vi "Debug - TCP - Write to Log File.vi"(9 "Transmission Log (or IP and Port String)":string, 10 "Flattened TCP Reference":string, 11 "Type of Write Opperation":T1) -> ()   [LabVIEW 2017, in "Communications Library.lvlib"]
doc: "Add a line to the TCP debug log file or modifys an already existing line to include the IP and Port number.\n\nWhen adding a new line, the placeholder should be used to mark the location where the IP and Port number will later be writte.\n\nNote: This VI must be non-reentrant, in order to avoid simulatenous writes to the same file by multiple threads."
uses:
  Communications Library.lvlib
  Typedefs/Debug - TCP Write Type--Enum.ctl
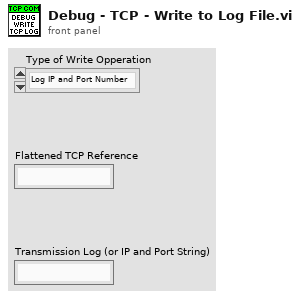
[diagram p1: front panel]
types:
  T1 = typedef "Communications Library.lvlib/Debug - TCP Write Type--Enum.ctl" = enum16{"Log IP and Port Number", "Append New Line"}
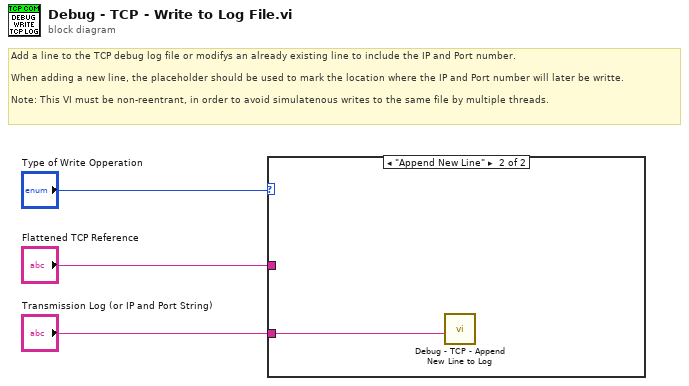
[diagram p0: block diagram]
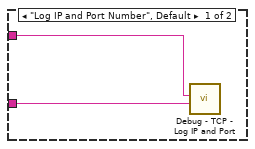
[diagram p2: hidden frame]
diagram:
  # "Add a line to the TCP debug log file or modifys an already existing line to include the IP and Port number.\n\nWhen adding a new line, the placeholder should be used to mark the location where the IP and Port number will later be writte.\n\nNote: This VI must be non-reentrant, in order to avoid simulatenous writes to the same file by multiple threads."
  n1 = case shown="\"Append New Line\"" "Type of Write Opperation" {
    tunnel: "Transmission Log (or IP and Port String)" -> [w4 w6]
    tunnel: "Flattened TCP Reference" -> [w5 _]
    frame "Log IP and Port Number", Default {
      n2 = call "Debug - TCP - Log IP and Port.vi"("IP and Port String"=w4, "Flattened TCP Reference"=w5) -> ()  [unwired: 10 in]
    }
    frame "Append New Line" {
      n3 = call "Debug - TCP - Append New Line to Log.vi"("Transmission Log"=w6) -> ()  [unwired: 11 in]
    }
  }
